vi "Pre Launch Init.vi"(11 "Nested in":refnum<class "Digital Acquisition.lvclass">) -> (0 "error out":errorcluster, 3 "Nested out":refnum<class "Digital Acquisition.lvclass">)   [LabVIEW 2020, in "Digital Acquisition.lvlib" / "Digital Acquisition.lvclass"]
doc: "(<B>Filename</B>: Actor Framework.lvlib:Actor.lvclass:Pre Launch Init.vi)\n\nDefines behavior that occurs after the Launch Nested Actor method is invoked but before the actor's Actor Core method begins running.\n\nBy default, this method does nothing. A descendant class may override it to define behavior."
uses:
  Digital Acquisition.lvclass
  Digital Acquisition.lvclass/Digital Acquisition.ctl
  <vilib>/ActorFramework/Actor/Actor.lvclass
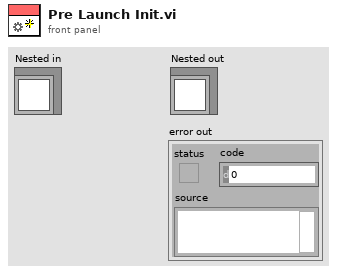
[diagram p1: front panel]
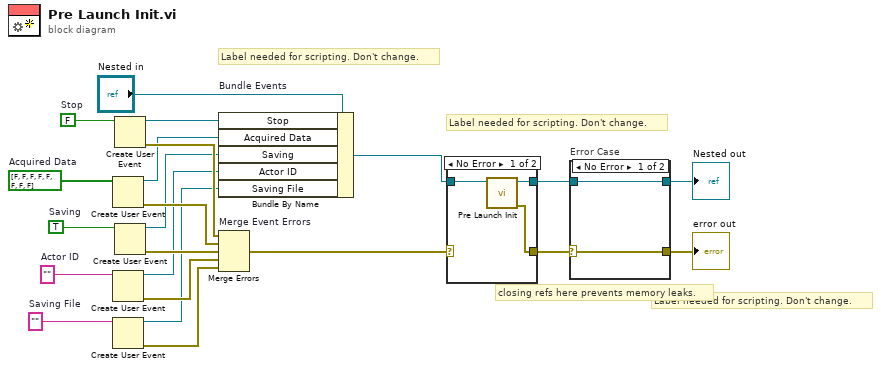
[diagram p0: block diagram]
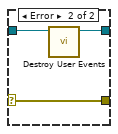
[diagram p3: hidden frame]
diagram:
  w4 = ""  # Saving File
  w5 = ""  # Actor ID
  w9 = TRUE  # Saving
  w12 = bool[] [FALSE, FALSE, FALSE, FALSE, FALSE, FALSE, FALSE, FALSE]  # Acquired Data
  w21 = FALSE  # Stop
  # "Label needed for scripting. Don't change."
  # "Label needed for scripting. Don't change."
  # "Label needed for scripting. Don't change."
  # "closing refs here prevents memory leaks."
  n1 = Create User Event(user event datatype=w12) -> (user event=w11:refnum<user-event>, error out=w10:errorcluster)  [unwired: 1 in]
  n2 = Create User Event(user event datatype=w5) -> (user event=w2:refnum<user-event>, error out=w7:errorcluster)  [unwired: 1 in]
  n3 = Create User Event(user event datatype=w4) -> (user event=w1:refnum<user-event>, error out=w6:errorcluster)  [unwired: 1 in]
  n4 = Create User Event(user event datatype=w21) -> (user event=w18:refnum<user-event>, error out=w20:errorcluster)  [unwired: 1 in]
  n5 = Create User Event(user event datatype=w9) -> (user event=w3:refnum<user-event>, error out=w8:errorcluster)  [unwired: 1 in]
  n6 = Bundle By Name "Bundle Events"(cluster="Nested in", "Stop"=w18, "Acquired Data"=w11, "Saving"=w3, "Actor ID"=w2, "Saving File"=w1) -> (w15:refnum<class "Digital Acquisition.lvclass">)
  n7 = Merge Errors "Merge Event Errors"(w20, w10, w8, w7, w6) -> (w14:errorcluster)
  n8 = case shown="No Error" w14 {
    selector: w14 -> [_ w27]
    tunnel: [w25 w26] -> w16
    tunnel: w15 -> [w24 w26]
    tunnel: [w23 w27] -> w13
    frame No Error {
      n9 = call-parent "Pre Launch Init.vi"("Actor in"=w24) -> ("error out"=w23:errorcluster, "Actor out"=w25:refnum<class "Digital Acquisition.lvclass">)  [unwired: 9 in]
    }
    frame Error {
    }
  }
  n10 = case "Error Case" shown="No Error" w13 {
    selector: w13 -> [w28 w32]
    tunnel: w16 -> [w29 w31]
    tunnel: [w29 w30] -> w19
    tunnel: [w28 w32] -> w17
    frame No Error {
    }
    frame Error {
      n11 = call "Destroy User Events.vi"("UI Template in"=w31) -> ("UI Template out"=w30:refnum<class "Digital Acquisition.lvclass">)  [unwired: 10 in]
    }
  }
  "error out" <- w17
  "Nested out" <- w19
